vi "Get Number Available Images.vi"(8 "error in (no error)":errorcluster, 10 "last":i32, 11 "first":i32) -> (0 "error out":errorcluster, 1 "function return":u32, 2 "last out":i32, 3 "first out":i32)   [LabVIEW 2014, in "atmcd32d.lvlib"]
doc: "unsigned int WINAPI GetNumberAvailableImages(at_32 * first, at_32 * last);"
uses:
  atmcd32d.lvlib
  atmcd32d.dll
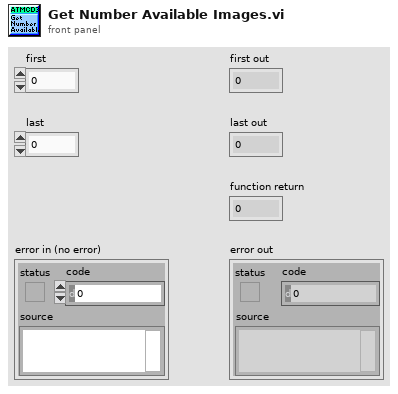
[diagram p1: front panel]
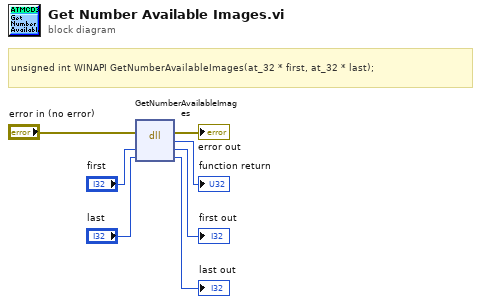
[diagram p0: block diagram]
diagram:
  # "unsigned int WINAPI GetNumberAvailableImages(at_32 * first, at_32 * last);"
  n1 = dll-call lib="C:/Users/Bakir/Documents/Lambda2-Testing/lib/Andorlib/atmcd32d.*" fn="GetNumberAvailableImages"(error in="error in (no error)", "first"="first", "last"="last") -> (error out=→"error out":errorcluster, →"function return":u32, "first"=→"first out":i32, "last"=→"last out":i32)  [unwired: 2 in, 1 out]
